vi "Introspection Input.vi"(8 "error in (no error)":errorcluster, 11 "ONNX Class in":refnum<class "ONNX Class.lvclass">) -> (0 "error out":errorcluster, 2 "Introspection Input":T1, 3 "ONNX Class out":refnum<class "ONNX Class.lvclass">)   [LabVIEW 2017, in "ONNX Class Library.lvlib" / "ONNX Class.lvclass"]
uses:
  ONNX Class.lvclass
  ONNX Class.lvclass/ONNX Class.ctl
  ONNX Class Library.lvlib
  TypeDef/IO.ctl
  TypeDef/Introspection.ctl
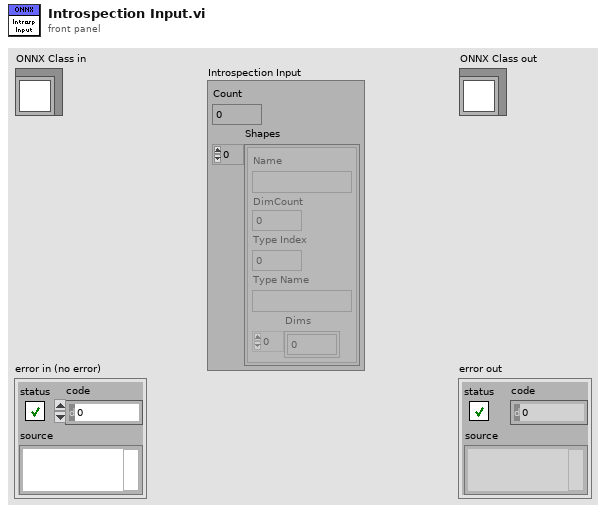
[diagram p1: front panel]
types:
  T1 = typedef "ONNX Class Library.lvlib/Introspection.ctl" = cluster{"Count":i32, "Shapes":T2[]}
  T2 = typedef "ONNX Class Library.lvlib/IO.ctl" = cluster{"Name":string, "DimCount":i32, "Type Index":i32, "Type Name":string, "Dims":i64[]}
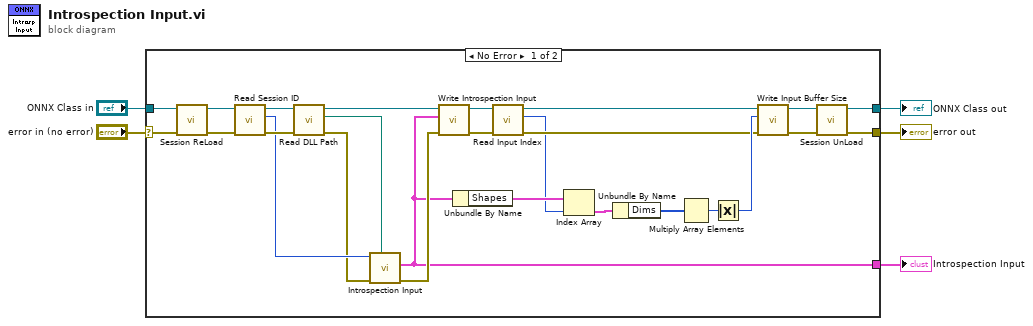
[diagram p0: block diagram]
diagram:
  n1 = case shown="No Error" "error in (no error)" {
    selector: "error in (no error)" -> [w29 w33]
    tunnel: [w19 w33] -> w4
    tunnel: [w20 w32] -> w2
    tunnel: "ONNX Class in" -> [w30 w32]
    tunnel: [w16 _] -> w1
    frame No Error {
      n2 = call-dynamic "Session ReLoad.vi"("error in (no error)"=w29, "ONNX Class in"=w30) -> ("error out"=w27:errorcluster, "ONNX Class out"=w28:refnum<class "ONNX Class.lvclass">)  [unwired: 8 in]
      n3 = call-dynamic "Read Session ID.vi"("error in (no error)"=w27, "ONNX Class in"=w28) -> ("error out"=w25:errorcluster, "Session ID"=w24:i32, "ONNX Class out"=w26:refnum<class "ONNX Class.lvclass">)  [unwired: 7 in]
      n4 = call-dynamic "Read DLL Path.vi"("error in (no error)"=w25, "ONNX Class in"=w26) -> ("error out"=w23:errorcluster, "DLL Path"=w22:path, "ONNX Class out"=w21:refnum<class "ONNX Class.lvclass">)  [unwired: 7 in]
      n5 = call "Introspection Input.vi"("DLL path"=w22, "error in (no error)"=w23, "session id in"=w24) -> ("error out"=w31:errorcluster, "Introspection Input"=w16:T1)  [unwired: 6 in, 1 out]
      n6 = call-dynamic "Write Introspection Input.vi"("error in (no error)"=w31, "Introspection"=w16, "ONNX Class in"=w21) -> ("error out"=w9:errorcluster, "ONNX Class out"=w10:refnum<class "ONNX Class.lvclass">)  [unwired: 7 in]
      n7 = Unbundle By Name(w16) -> ("Shapes"=w15:T2[])
      n8 = call-dynamic "Read Input Index.vi"("error in (no error)"=w9, "ONNX Class in"=w10) -> ("error out"=w7:errorcluster, "Input Index"=w6:i32, "ONNX Class out"=w8:refnum<class "ONNX Class.lvclass">)  [unwired: 7 in]
      n9 = Index Array(array=w15, index=w6) -> (element=w14:T2)
      n10 = Unbundle By Name(w14) -> ("Dims"=w13:i64[])
      n11 = Multiply Array Elements(1:w13) -> (0:w12:i64)
      n12 = Absolute Value(x=w12) -> (abs(x)=w11:i64)
      n13 = call-dynamic "Write Input Buffer Size.vi"("error in (no error)"=w7, "Input Buffer Size"=w11, "ONNX Class in"=w8) -> ("error out"=w17:errorcluster, "ONNX Class out"=w18:refnum<class "ONNX Class.lvclass">)  [unwired: 7 in]
      n14 = call-dynamic "Session UnLoad.vi"("error in (no error)"=w17, "ONNX Class in"=w18) -> ("error out"=w19:errorcluster, "ONNX Class out"=w20:refnum<class "ONNX Class.lvclass">)  [unwired: 8 in]
    }
    frame Error {
    }
  }
  "error out" <- w4
  "ONNX Class out" <- w2
  "Introspection Input" <- w1
